vi "Read MotorManager.vi"(8 "error in (no error)":errorcluster, 11 "ICS in":refnum<class "ICS.lvclass">) -> (0 "error out":errorcluster, 2 "MotorManager.lvclass":refnum<class "MotorManager.lvclass">, 3 "ICS out":refnum<class "ICS.lvclass">)   [LabVIEW 2018, in "ICS.lvclass"]
uses:
  ICS.lvclass
  MotorManager/MotorManager.lvclass
  ICS.lvclass/ICS.ctl
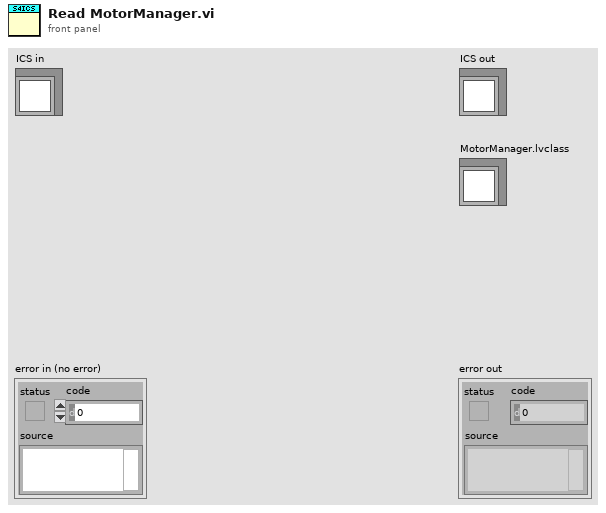
[diagram p1: front panel]
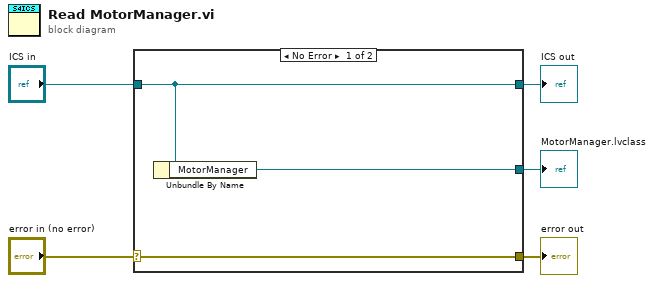
[diagram p0: block diagram]
diagram:
  n1 = case shown="No Error" "error in (no error)" {
    selector: "error in (no error)" -> [w8 w9]
    tunnel: [w8 w9] -> w4
    tunnel: [w7 w10] -> w2
    tunnel: "ICS in" -> [w7 w10]
    tunnel: [w6 _] -> w1
    frame No Error {
      n2 = Unbundle By Name(w7) -> ("MotorManager"=w6:refnum<class "MotorManager.lvclass">)
    }
    frame Error {
    }
  }
  "error out" <- w4
  "ICS out" <- w2
  "MotorManager.lvclass" <- w1
